vi "calculate edge fit 4x.vi"(8 "error in (no error)":errorcluster, 11 "LineCCD in":refnum<class "LineCCD.lvclass">) -> (0 "error out":errorcluster, 3 "LineCCD out":refnum<class "LineCCD.lvclass">)   [LabVIEW 2012, in "LineCCD.lvclass"]
uses:
  LineCCD.lvclass
  LineCCD.lvclass/LineCCD.ctl
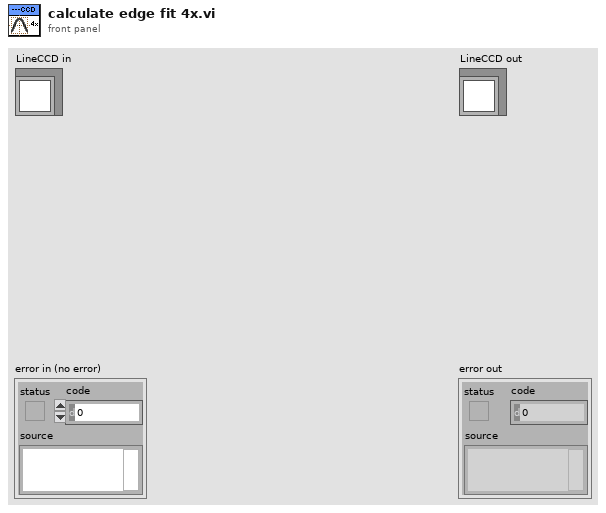
[diagram p1: front panel]
types:
  T1 = typedef "LineCCD.lvclass/fitting parameters.ctl" = cluster{"y_min":dbl, "y_mean":dbl, "A_g":dbl, "STD":dbl, "x_0":dbl}
  T2 = cluster{"best fit parameters[0]":dbl, "best fit parameters[1]":dbl, "best fit parameters[2]":dbl, "best fit parameters[3]":dbl, "best fit parameters[4]":dbl}
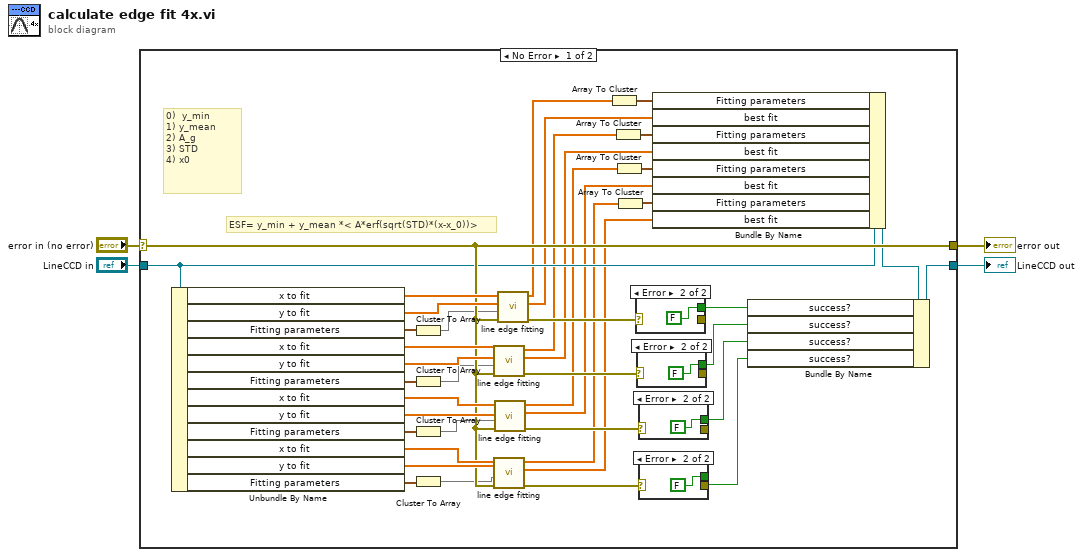
[diagram p0: block diagram]
diagram:
  n1 = case shown="No Error" "error in (no error)" {
    selector: "error in (no error)" -> [w27 w54]
    tunnel: [w27 w54] -> w3
    tunnel: [w32 w53] -> w1
    tunnel: "LineCCD in" -> [w26 w53]
    frame No Error {
      # "0)  y_min\n1) y_mean\n2) A_g\n3) STD\n4) x0"
      # "ESF= y_min + y_mean *< A*erf(sqrt(STD)*(x-x_0))>"
      n2 = Unbundle By Name(w26) -> ("x to fit"=w44:dbl[], "y to fit"=w43:dbl[], "Fitting parameters"=w20:T1, "x to fit"=w42:dbl[], "y to fit"=w41:dbl[], "Fitting parameters"=w18:T1, "x to fit"=w40:dbl[], "y to fit"=w39:dbl[], "Fitting parameters"=w16:T1, "x to fit"=w38:dbl[], "y to fit"=w37:dbl[], "Fitting parameters"=w14:T1)
      n3 = Cluster To Array(cluster=w20) -> (array=w19:dbl[])
      n4 = Cluster To Array(cluster=w18) -> (array=w17:dbl[])
      n5 = Cluster To Array(cluster=w16) -> (array=w15:dbl[])
      n6 = Cluster To Array(cluster=w14) -> (array=w13:dbl[])
      n7 = call "line edge fitting.vi"("error in (no error)"=w27, "Paramter guess"=w17, "y"=w41, "x"=w42) -> ("error out"=w35:errorcluster, "best nonlinear fit"=w22:dbl[], "best fit parameters"=w9:dbl[])  [unwired: 4 in, 1 out]
      n8 = call "line edge fitting.vi"("error in (no error)"=w27, "Paramter guess"=w13, "y"=w37, "x"=w38) -> ("error out"=w33:errorcluster, "best nonlinear fit"=w24:dbl[], "best fit parameters"=w5:dbl[])  [unwired: 4 in, 1 out]
      n9 = call "line edge fitting.vi"("error in (no error)"=w27, "Paramter guess"=w15, "y"=w39, "x"=w40) -> ("error out"=w34:errorcluster, "best nonlinear fit"=w23:dbl[], "best fit parameters"=w7:dbl[])  [unwired: 4 in, 1 out]
      n10 = call "line edge fitting.vi"("error in (no error)"=w27, "Paramter guess"=w19, "y"=w43, "x"=w44) -> ("error out"=w36:errorcluster, "best nonlinear fit"=w21:dbl[], "best fit parameters"=w11:dbl[])  [unwired: 4 in, 1 out]
      n11 = Array To Cluster(array=w11) -> (cluster=w12:T2)
      n12 = Array To Cluster(array=w9) -> (cluster=w10:T2)
      n13 = Array To Cluster(array=w7) -> (cluster=w8:T2)
      n14 = Array To Cluster(array=w5) -> (cluster=w6:T2)
      n15 = case shown="Error" w36 {
        selector: w36 -> [w51 _]
        tunnel: [w51 _] -> _
        tunnel: [_ FALSE] -> w31
        frame No Error {
        }
        frame Error {
        }
      }
      n16 = case shown="Error" w35 {
        selector: w35 -> [w49 _]
        tunnel: [w49 _] -> _
        tunnel: [_ FALSE] -> w30
        frame No Error {
        }
        frame Error {
        }
      }
      n17 = case shown="Error" w34 {
        selector: w34 -> [w47 _]
        tunnel: [w47 _] -> _
        tunnel: [_ FALSE] -> w29
        frame No Error {
        }
        frame Error {
        }
      }
      n18 = case shown="Error" w33 {
        selector: w33 -> [w45 _]
        tunnel: [w45 _] -> _
        tunnel: [_ FALSE] -> w28
        frame No Error {
        }
        frame Error {
        }
      }
      n19 = Bundle By Name(cluster=w26, "Fitting parameters"=w12, "best fit"=w21, "Fitting parameters"=w10, "best fit"=w22, "Fitting parameters"=w8, "best fit"=w23, "Fitting parameters"=w6, "best fit"=w24) -> (w25:refnum<class "LineCCD.lvclass">)
      n20 = Bundle By Name(cluster=w25, "success?"=w31, "success?"=w30, "success?"=w29, "success?"=w28) -> (w32:refnum<class "LineCCD.lvclass">)
    }
    frame Error {
    }
  }
  "error out" <- w3
  "LineCCD out" <- w1
